vi "Initialize Alicat.vi"(8 "error in":errorcluster, 11 "Alicat Device In":refnum<class "Alicat Device.lvclass">) -> (0 "error out":errorcluster, 3 "Alicat Device Out":refnum<class "Alicat Device.lvclass">)   [LabVIEW 2015, in "Alicat Device.lvclass"]
doc: "Configure the serial port for communication with the Alicat devices. We will create new Alicat objects based upon an input array of addresses. If an address is no good, then we will delete the session reference and move onto the next address. We determine if the session is good by sending a request for data to the device until the device \"wakes up\" and responds properly. If the device does not repsond properly, then set the boolean property <b>Active</b> to alert potential callers that this instantiation is non-communicative.\n\nAlthough the caller can configure the port with the desired serial and message settings, the default settings should be sufficient for most applications."
uses:
  Alicat Device.lvclass
  Configurable Device/Configurable Device.lvclass/Configurable Device.ctl
  Reusable/Session APIs/File Access/Config Data/Config Data.lvclass/Config Data.ctl
  Alicat Device.lvclass/Alicat Device.ctl
  Reusable/Session APIs/Serial/Serial Session.lvclass
  Accessors/Read Session Handle.vi
  Configurable Device/Read Handle.vi
  <vilib>/Utility/config.llb/Read Key (String).vi
  <vilib>/Utility/config.llb/Read Key (Double).vi
  <vilib>/Utility/config.llb/Read Key (Boolean).vi
  Reusable/Session APIs/File Access/Config Data/Config Data.lvclass
  <userlib>/_Session Fwk/Session - Root.lvclass
  <vilib>/Utility/config.llb/NI_LVConfig.lvlib
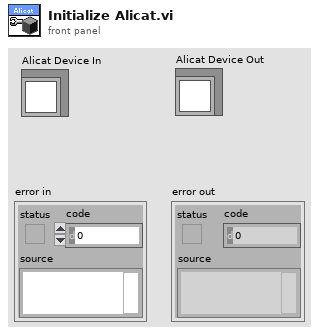
[diagram p1: front panel]
types:
  T1 = typedef "Config Data.lvclass/Config Session.ctl" = refnum<data-value>
  T2 = typedef "NI_LVConfig.lvlib/Config Data RefNum.ctl" = refnum<k1>
  T3 = typedef "Session - Root.lvclass/Session Handle.ctl" = refnum<data-value>
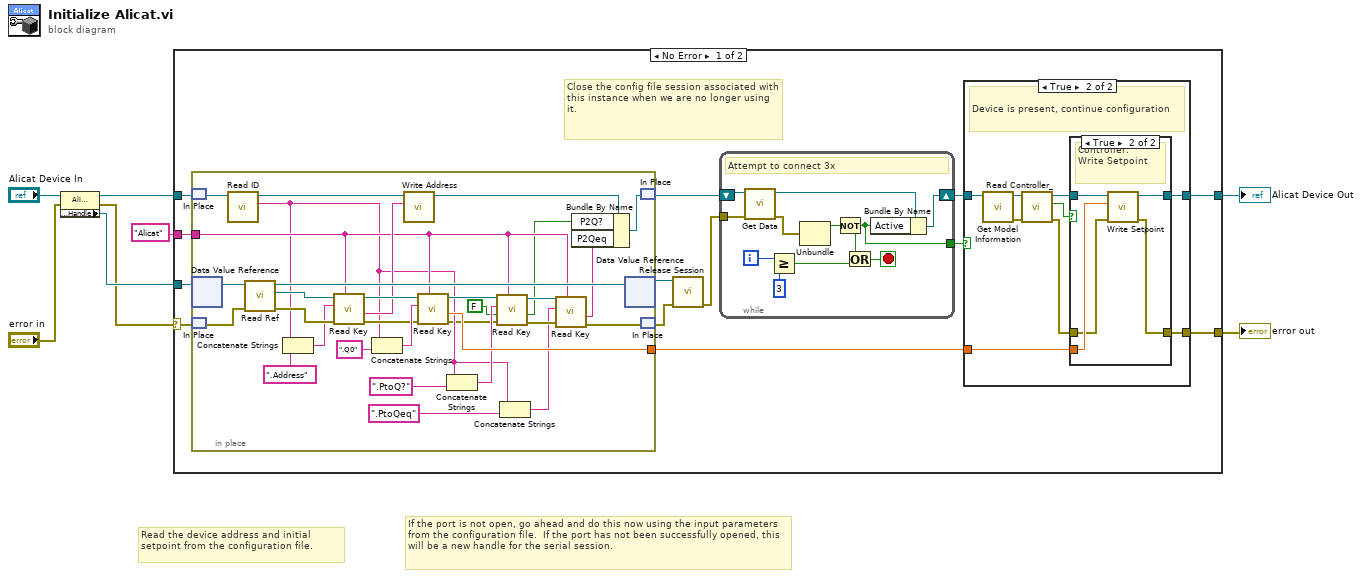
[diagram p0: block diagram]
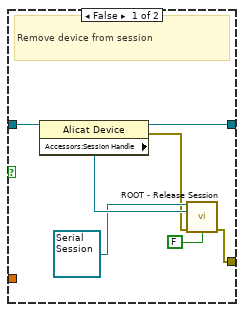
[diagram p2: hidden frame]
diagram:
  # "If the port is not open, go ahead and do this now using the input parameters from the configuration file.  If the port has not been successfully opened, this will be a new handle for the serial session."
  # "Read the device address and initial setpoint from the configuration file."
  n1 = property class="Alicat Device"(reference="Alicat Device In", error in="error in") -> (reference out=w3:refnum<class "Alicat Device.lvclass">, error out=w6:errorcluster, "Accessors:Handle"=w7:T1)
  n2 = case shown="No Error" w6 {
    selector: w6 -> [w10 w87]
    tunnel: w7 -> [w21 _]
    tunnel: "Alicat" ("section") -> [w20 _]
    tunnel: [w18 w87] -> w1
    tunnel: [w15 w88] -> w2
    tunnel: w3 -> [w11 w88]
    frame No Error {
      # "Close the config file session associated with this instance when we are no longer using it."
      n3 = in-place {
        in-place-border: w20 -> [w65]
        in-place-border: [w72] -> w16
        n4 = in-place-match #1(w11) -> (w75:refnum<class "Alicat Device.lvclass">)
        n5 = in-place-dvr #2(w21) -> (w86:refnum<class "Config Data.lvclass">)  [unwired: 1 out]
        n6 = in-place-match #3(w10) -> (w85:errorcluster)
        n7 = call "Read ID.vi"("Alicat Device in"=w75) -> ("ID"=w64:string, "Alicat Device out"=w74:refnum<class "Alicat Device.lvclass">)  [unwired: 8 in, 1 out]
        n8 = call "Read Ref.vi"("error in (no error)"=w85, "Config Data in"=w86) -> ("error out"=w83:errorcluster, "config data"=w84:T2, "Config Data out"=w76:refnum<class "Config Data.lvclass">)  [unwired: 7 in]
        n9 = Concatenate Strings(w64, ".Address" ("string")) -> (w81:string)
        n10 = call-poly <vilib>:"Read Key.vi"("section"=w65, "error in (no error)"=w83, "key"=w81, "refnum"=w84) -> ("error out"=w77:errorcluster, "value"=w73:string, "refnum out"=w80:T2)  [unwired: 4 in, 1 out]
        n11 = Concatenate Strings(w64, ".Q0" ("string")) -> (w78:string)
        n12 = call "Write Address.vi"("Address"=w73, "Alicat Device in"=w74) -> ("Alicat Device out"=w61:refnum<class "Alicat Device.lvclass">)  [unwired: 8 in, 1 out]
        n13 = call-poly <vilib>:"Read Key.vi"("section"=w65, "error in (no error)"=w77, "key"=w78, "refnum"=w80) -> ("error out"=w57:errorcluster, "value"=w72:dbl, "refnum out"=w71:T2)  [unwired: 4 in, 1 out]
        n14 = Concatenate Strings(w64, ".PtoQ?" ("string")) -> (w69:string)
        n15 = call-poly <vilib>:"Read Key.vi"("section"=w65, "error in (no error)"=w57, "default value"=FALSE, "key"=w69, "refnum"=w71) -> ("error out"=w66:errorcluster, "value"=w60:bool, "refnum out"=w67:T2)  [unwired: 3 in, 1 out]
        n16 = Concatenate Strings(w64, ".PtoQeq" ("string")) -> (w62:string)
        n17 = call-poly <vilib>:"Read Key.vi"("section"=w65, "error in (no error)"=w66, "key"=w62, "refnum"=w67) -> ("error out"=w56:errorcluster, "value"=w59:string)  [unwired: 4 in, 2 out]
        n18 = Bundle By Name(cluster=w61, "P2Q?"=w60, "P2Qeq"=w59) -> (w58:refnum<class "Alicat Device.lvclass">)
        n19 = in-place-dvr #2(w76) -> (w14:T1)  [unwired: 1 out]
        n20 = in-place-match #1(w58) -> (w19:refnum<class "Alicat Device.lvclass">)
        n21 = in-place-match #3(w56) -> (w13:errorcluster)
      }
      n22 = call "Release Session.vi"("error in"=w13, "Session Handle"=w14) -> ("error out"=w12:errorcluster)  [unwired: 8 in, 1 out]
      n23 = while {
        tunnel: w12 -> [w50]
        shift-right: [w48] -> w17
        shift-left: w19 -> [w51]
        tunnel: [w47] -> w9
        i -> [w45]
        stop <- w52 stop-if-true
        # "Attempt to connect 3x"
        n24 = call-dynamic "Get Data.vi"("error in"=w50, "Cfg Dev in"=w51) -> ("error out"=w46:errorcluster, "Cfg Dev out"=w49:refnum<class "Alicat Device.lvclass">)  [unwired: 7 in, 1 out]
        n25 = Greater Or Equal?(x=w45, y=3) -> (x >= y?=w54:bool)
        n26 = Unbundle(w46) -> ("status"=w53:bool)  [unwired: 2 out]
        n27 = Not(x=w53) -> (.not. x?=w47:bool)
        n28 = Or(x=w47, y=w54) -> (x .or. y?=w52:bool)
        n29 = Bundle By Name(cluster=w49, "Active"=w47) -> (w48:refnum<class "Alicat Device.lvclass">)
      }
      n30 = case shown="True" w9 {
        tunnel: [w24 w30] -> w18
        tunnel: w17 -> [w28 w37]
        tunnel: w16 -> [_ w31]
        tunnel: [w27 w29] -> w15
        frame False {
          # "Remove device from session"
          n31 = property class="Alicat Device"(reference=w28) -> (reference out=w27:refnum<class "Alicat Device.lvclass">, error out=w23:errorcluster, "Accessors:Session Handle"=w26:T3)  [unwired: 1 in]
          n32 = call <userlib>:"ROOT - Release Session.vi"("OBJ - Session in"=refnum<class "Serial Session.lvclass"> refnum ("Serial Session in"), "Session Handle in"=w26, "error in (no error)"=w23, "force destroy? (F)"=FALSE) -> ("error out"=w24:errorcluster)  [unwired: 10 in, 1 out]
        }
        frame True {
          # "Device is present, continue configuration"
          n33 = call "Get Model Information.vi"("Alicat Device in"=w37) -> ("error out"=w35:errorcluster, "Alicat Device out"=w36:refnum<class "Alicat Device.lvclass">)  [unwired: 8 in, 1 out]
          n34 = call "Read Controller_.vi"("error in"=w35, "Alicat Device in"=w36) -> ("error out"=w33:errorcluster, "Controller?"=w34:bool, "Alicat Device out"=w32:refnum<class "Alicat Device.lvclass">)  [unwired: 7 in]
          n35 = case shown="True" w34 {
            tunnel: w33 -> [w38 w42]
            tunnel: w32 -> [w39 w44]
            tunnel: w31 -> [_ w43]
            tunnel: [w38 w41] -> w30
            tunnel: [w39 w40] -> w29
            frame False {
            }
            frame True {
              # "Controller:\nWrite Setpoint"
              n36 = call "Write Setpoint.vi"("error in"=w42, "Setpoint"=w43, "Alicat Device in"=w44) -> ("error out"=w41:errorcluster, "Alicat Device out"=w40:refnum<class "Alicat Device.lvclass">)  [unwired: 6 in, 1 out]
            }
          }
        }
      }
    }
    frame Error {
    }
  }
  "error out" <- w1
  "Alicat Device Out" <- w2
